vi "+S2C_IMAGE_Process.vi"(8 "Error In":errorcluster) -> (0 "Error Out":errorcluster)   [LabVIEW 2015]
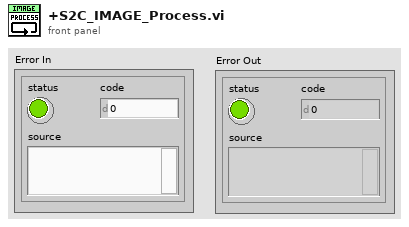
[diagram p1: front panel]
types:
  T1 = cluster{"Caller-Q":refnum<queue>, "Command":string, "Return":string, "Data":variant, "Timeout":dbl}
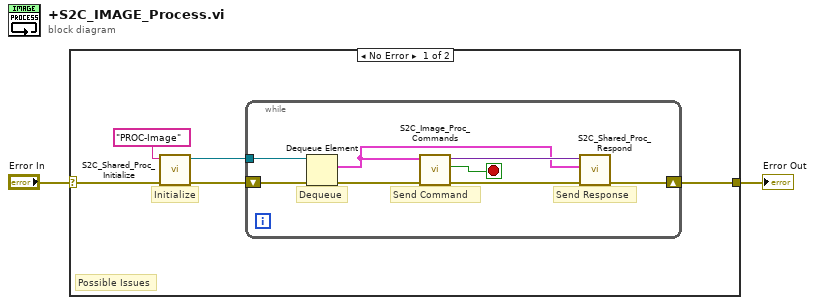
[diagram p0: block diagram]
diagram:
  n1 = case shown="No Error" "Error In" {
    selector: "Error In" -> [w6 w16]
    tunnel: [w7 w16] -> w1
    frame No Error {
      # "Possible Issues"
      # "Initialize"
      n2 = call "S2C_Shared_Proc_Initialize.vi"("Error In"=w6, "Q-Name"="PROC-Image" ("name (unnamed)")) -> ("Error Out"=w5:errorcluster, "Q-Ref"=w4:refnum<queue>)  [unwired: 8 in]
      n3 = while {
        shift-right: [w13] -> w7
        shift-left: w5 -> [w15]
        tunnel: w4 -> [w14]
        stop <- w9 stop-if-true
        # "Send Command"
        # "Send Response"
        # "Dequeue"
        n4 = Dequeue Element(queue=w14, error in (no error)=w15) -> (element=w8:T1, error out=w12:errorcluster)  [unwired: 1 in, 2 out]
        n5 = call "S2C_Image_Proc_Commands.vi"("Error In"=w12, "Settings"=w8) -> ("Error Out"=w10:errorcluster, "Stop?"=w9:bool, "Response"=w11:variant)  [unwired: 7 in]
        n6 = call "S2C_Shared_Proc_Respond.vi"("Error In"=w10, "Settings"=w8, "Response"=w11) -> ("Error Out"=w13:errorcluster)  [unwired: 8 in]
      }
    }
    frame Error {
    }
  }
  "Error Out" <- w1
